vi "Elevation to Pressure.vi"(1 "Elevation [ft]":dbl) -> (0 "Pressure [psia]":dbl)   [LabVIEW 2020]
uses:
  <vilib>/gmath/NI_Gmath.lvlib
panel:
  in  "ElevationToPressure":dbl[][](array[numeric])=[[-1500.0, 15.51026974], [-1000.0, 15.23488864], [-500.0, 14.96348006], [0.0, 14.696], [500.0, 14.43240481], [1000.0, 14.17265118], [1500.0, 13.91669613], [2000.0, 13.66449702], [2500.0, 13.41601153], [3000.0, 13.17119769], [3500.0, 12.93001384], [4000.0, 12.69241866], [4500.0, 12.45837117], [5000.0, 12.22783068], [5500.0, 12.00075687], [6000.0, 11.77710969], [6500.0, 11.55684946], [7000.0, 11.3399368]]
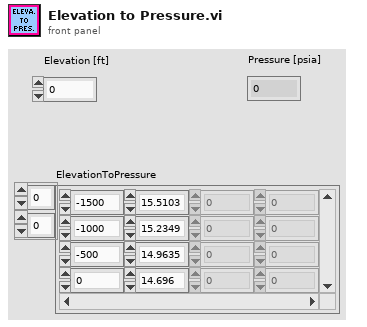
[diagram p1: front panel]
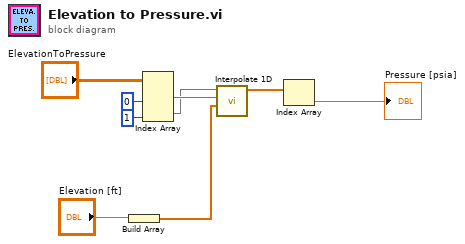
[diagram p0: block diagram]
diagram:
  n1 = Build Array("Elevation [ft]") -> (w4:dbl[])
  n2 = Index Array(array="ElevationToPressure", index (col) #1=0 ("disabled index (col)"), index (col) #2=1 ("index (col)")) -> (element #1=w6:dbl[], element #2=w3:dbl[])  [unwired: 2 in]
  n3 = call <vilib>:"Interpolate 1D.vi"("xi"=w4, "X"=w6, "Y"=w3) -> ("yi"=w2:dbl[])  [unwired: 6 in, 2 out]
  n4 = Index Array(array=w2) -> (element=→"Pressure [psia]":dbl)  [unwired: 1 in]
